vi "SeCrTs-Irms_Module_A.vi"(7 "Data FIFO Ref":T1, 8 "error in":errorcluster, 11 "TCP Network Connection in":refnum<k5>) -> (0 "error out":errorcluster, 3 "TCP Network Connection out":refnum<k5>)   [LabVIEW 2022 SP3]
uses:
  RT Controls/SeCrTs-Data FIFO.ctl
  <vilib>/Analysis/3filter.llb/Filter Passband Type.ctl
  RT Controls/SeCrTs-FGV Read write.ctl
  <vilib>/Analysis/NI_AALBase.lvlib
  <vilib>/ptbypt/NI_PtbyPt.lvlib
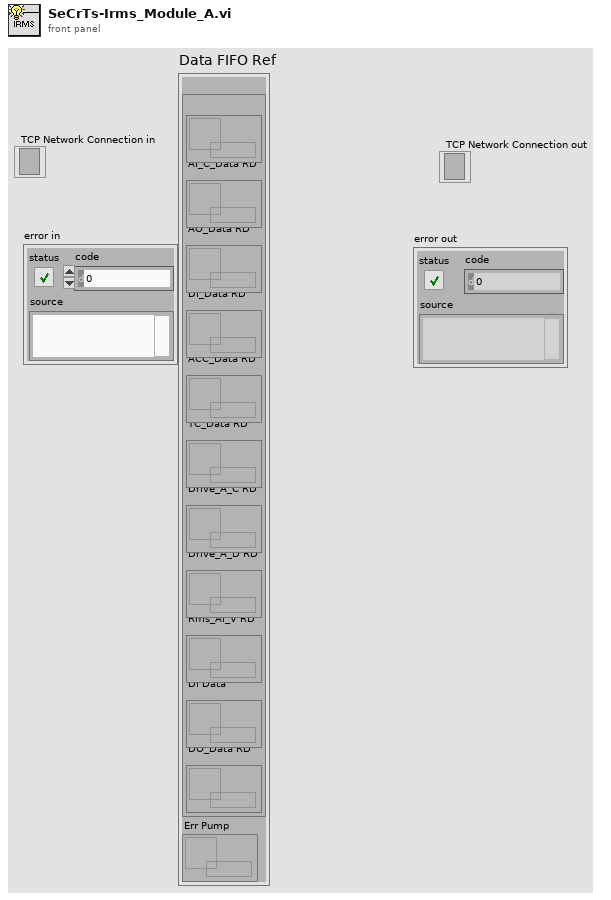
[diagram p1: front panel]
types:
  T1 = typedef "SeCrTs-Data FIFO.ctl" = cluster{"RD":cluster{"AI_V_Data RD":refnum<queue>, "AI_C_Data RD":refnum<queue>, "AO_Data RD":refnum<queue>, "DI_Data RD":refnum<queue>, "ACC_Data RD":refnum<queue>, "TC_Data RD":refnum<queue>, "Drive_A_C RD":refnum<queue>, "Drive_A_D RD":refnum<queue>, "Rms_AI_V RD":refnum<queue>, "DI Data":refnum<queue>, "DO_Data RD":refnum<queue>}, "Err Pump":refnum<queue>}
  T2 = typedef "SeCrTs-FGV Read write.ctl" = enum16{"Write", "Read"}
  T3 = typedef "NI_AALBase.lvlib/Filter Passband Type.ctl" = enum32{"Lowpass", "Highpass", "Bandpass", "Bandstop"}
  T4 = cluster{"En_Drive_A":bool, "En_Drive_L":bool, "Exit_Drive_A":bool, "Exit_Drive_L":bool}
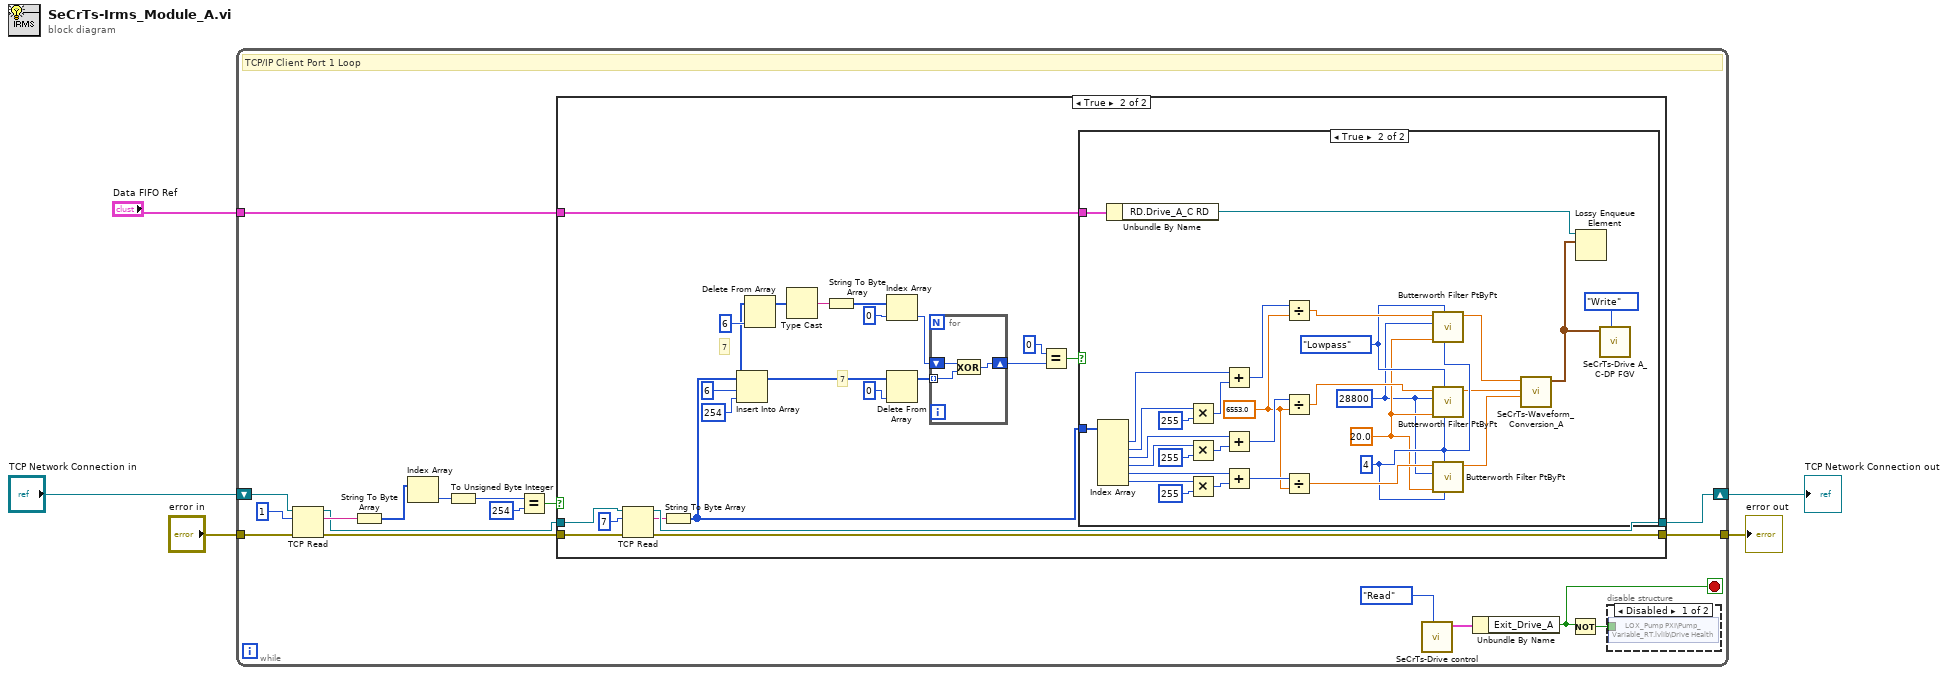
[diagram p0: block diagram]
diagram:
  n1 = while {
    tunnel: [w15] -> w3
    shift-right: [w14] -> w4
    shift-left: "TCP Network Connection in" -> [w23]
    tunnel: "error in" -> [w11]
    tunnel: "Data FIFO Ref" -> [w6]
    stop <- w8 stop-if-true
    # "TCP/IP Client Port 1 Loop"
    n2 = TCP Read(connection ID=w23, bytes to read=1, error in (no error)=w11) -> (connection ID out=w16:refnum<k5>, data out=w17:string, error out=w12:errorcluster)  [unwired: 2 in]
    n3 = String To Byte Array(string=w17) -> (unsigned byte array=w21:u8[])
    n4 = Index Array(array=w21) -> (element=w20:u8)  [unwired: 1 in]
    n5 = To Unsigned Byte Integer(number=w20) -> (unsigned 8bit integer=w19:u8)
    n6 = Equal?(x=w19, y=u8 254) -> (x = y?=w13:bool)
    n7 = case shown="True" w13 {
      tunnel: w16 -> [w25 w48]
      tunnel: w12 -> [w26 w47]
      tunnel: [w26 w46] -> w15
      tunnel: [w25 w45] -> w14
      tunnel: w6 -> [_ w27]
      frame False {
      }
      frame True {
        # "7"
        # "7"
        n8 = TCP Read(connection ID=w48, bytes to read=7, error in (no error)=w47) -> (connection ID out=w45:refnum<k5>, data out=w44:string, error out=w46:errorcluster)  [unwired: 2 in]
        n9 = String To Byte Array(string=w44) -> (unsigned byte array=w31:u8[])
        n10 = Insert Into Array(array=w31, index=6, new element=u8 254 ("new element/subarray")) -> (w32:u8[])
        n11 = Delete From Array(array=w31, index=6) -> (array with subset deleted=w35:u8[])  [unwired: 1 in, 1 out]
        n12 = Type Cast(x=w35) -> (*(type *) &x=w41:string)  [unwired: 1 in]
        n13 = String To Byte Array(string=w41) -> (unsigned byte array=w36:u8[])
        n14 = Index Array(array=w36, index=0) -> (element=w39:u8)
        n15 = Delete From Array(array=w32, index=0) -> (array with subset deleted=w38:u8[])  [unwired: 1 in, 1 out]
        n16 = for {
          shift-right: [w81] -> w29
          shift-left: w39 -> [w82]
          tunnel: w38 -> [w80] mode=indexing
          n17 = Exclusive Or(1:w80, 2:w82) -> (0:w81:u8)
        }
        n18 = Equal?(x=u8 0, y=w29) -> (x = y?=w28:bool)
        n19 = case shown="True" w28 {
          tunnel: w31 -> [_ w64]
          tunnel: w27 -> [_ w52]
          frame False {
          }
          frame True {
            w59 = Filter_Passband_Type."Lowpass" ("filter type")
            w58 = 4 ("order")
            w57 = 20.0 ("low cutoff freq: fl")
            w56 = 28800 ("rank")
            w63 = 6553.0
            n20 = Index Array(array=w64) -> (element #1=w77:u8, element #2=w76:u8, element #3=w71:u8, element #4=w70:u8, element #5=w69:u8, element #6=w68:u8)  [unwired: 6 in]
            n21 = Unbundle By Name(w52) -> ("RD.Drive_A_C RD"=w51:refnum<queue>)
            n22 = Multiply(x=w76, y=u32 255) -> (x*y=w78:u32)
            n23 = Multiply(x=w70, y=u32 255) -> (x*y=w75:u32)
            n24 = Multiply(x=w68, y=u32 255) -> (x*y=w72:u32)
            n25 = Add(x=w77, y=w78) -> (x+y=w67:u32)
            n26 = Add(x=w71, y=w75) -> (x+y=w66:u32)
            n27 = Add(x=w69, y=w72) -> (x+y=w65:u32)
            n28 = Divide(x=w67, y=w63) -> (x/y=w62:dbl)
            n29 = Divide(x=w66, y=w63) -> (x/y=w61:dbl)
            n30 = Divide(x=w65, y=w63) -> (x/y=w60:dbl)
            n31 = call <vilib>:"Butterworth Filter PtByPt.vi"("order"=w58, "filter type"=w59, "low cutoff freq: fl"=w57, "sampling freq: fs"=w56, "x"=w62) -> ("Filtered x"=w55:dbl)  [unwired: 4 in, 1 out]
            n32 = call <vilib>:"Butterworth Filter PtByPt.vi"("order"=w58, "filter type"=w59, "low cutoff freq: fl"=w57, "sampling freq: fs"=w56, "x"=w61) -> ("Filtered x"=w54:dbl)  [unwired: 4 in, 1 out]
            n33 = call <vilib>:"Butterworth Filter PtByPt.vi"("order"=w58, "filter type"=w59, "low cutoff freq: fl"=w57, "sampling freq: fs"=w56, "x"=w60) -> ("Filtered x"=w53:dbl)  [unwired: 4 in, 1 out]
            n34 = call "SeCrTs-Waveform_Conversion_A.vi"("Irms3"=w53, "Irms2"=w54, "Irms1"=w55) -> ("Array"=w49:waveform(dbl)[])  [unwired: 8 in]
            n35 = Lossy Enqueue Element(queue=w51, element=w49) -> ()  [unwired: 1 in, 4 out]
            n36 = call "SeCrTs-Drive A_C-DP FGV.vi"("Write/Read"=SeCrTs-FGV_Read_write."Write", "Drive A_C"=w49) -> ()  [unwired: 8 in, 2 out]
          }
        }
      }
    }
    n37 = call "SeCrTs-Drive control.vi"("Action"=enum16{"Init", "Write", "Read"}."Read") -> ("Loop Control Out"=w9:T4)  [unwired: 9 in, 1 out]
    n38 = Unbundle By Name(w9) -> ("Exit_Drive_A"=w8:bool)
    n39 = Not(x=w8) -> (.not. x?=w10:bool)
    n40 = disable-structure shown="Disabled" {
      disable-tunnel: w10 -> [w24 _]
      frame Disabled {
        n41 = shared-variable "LOX_Pump PXI\\Pump_Variable_RT.lvlib\\Drive Health"(w24) -> ()  [unwired: 1 in, 1 out]
      }
      frame Enabled {
      }
    }
  }
  "TCP Network Connection out" <- w4
  "error out" <- w3
